vi "WAIT.vi"(7 "arguments":string[](array[string]), 9 "Reinit":bool, 10 "HMI to Control":T1, 11 "SensorInputData":T2) -> (1 "Done":bool, 2 "SensorInputDataOut":T2, 3 "HMI to Control Out":T1)   [LabVIEW 2015]
uses:
  Typedefs/SensorInputData.ctl
  Typedefs/HMI_to_Control.ctl
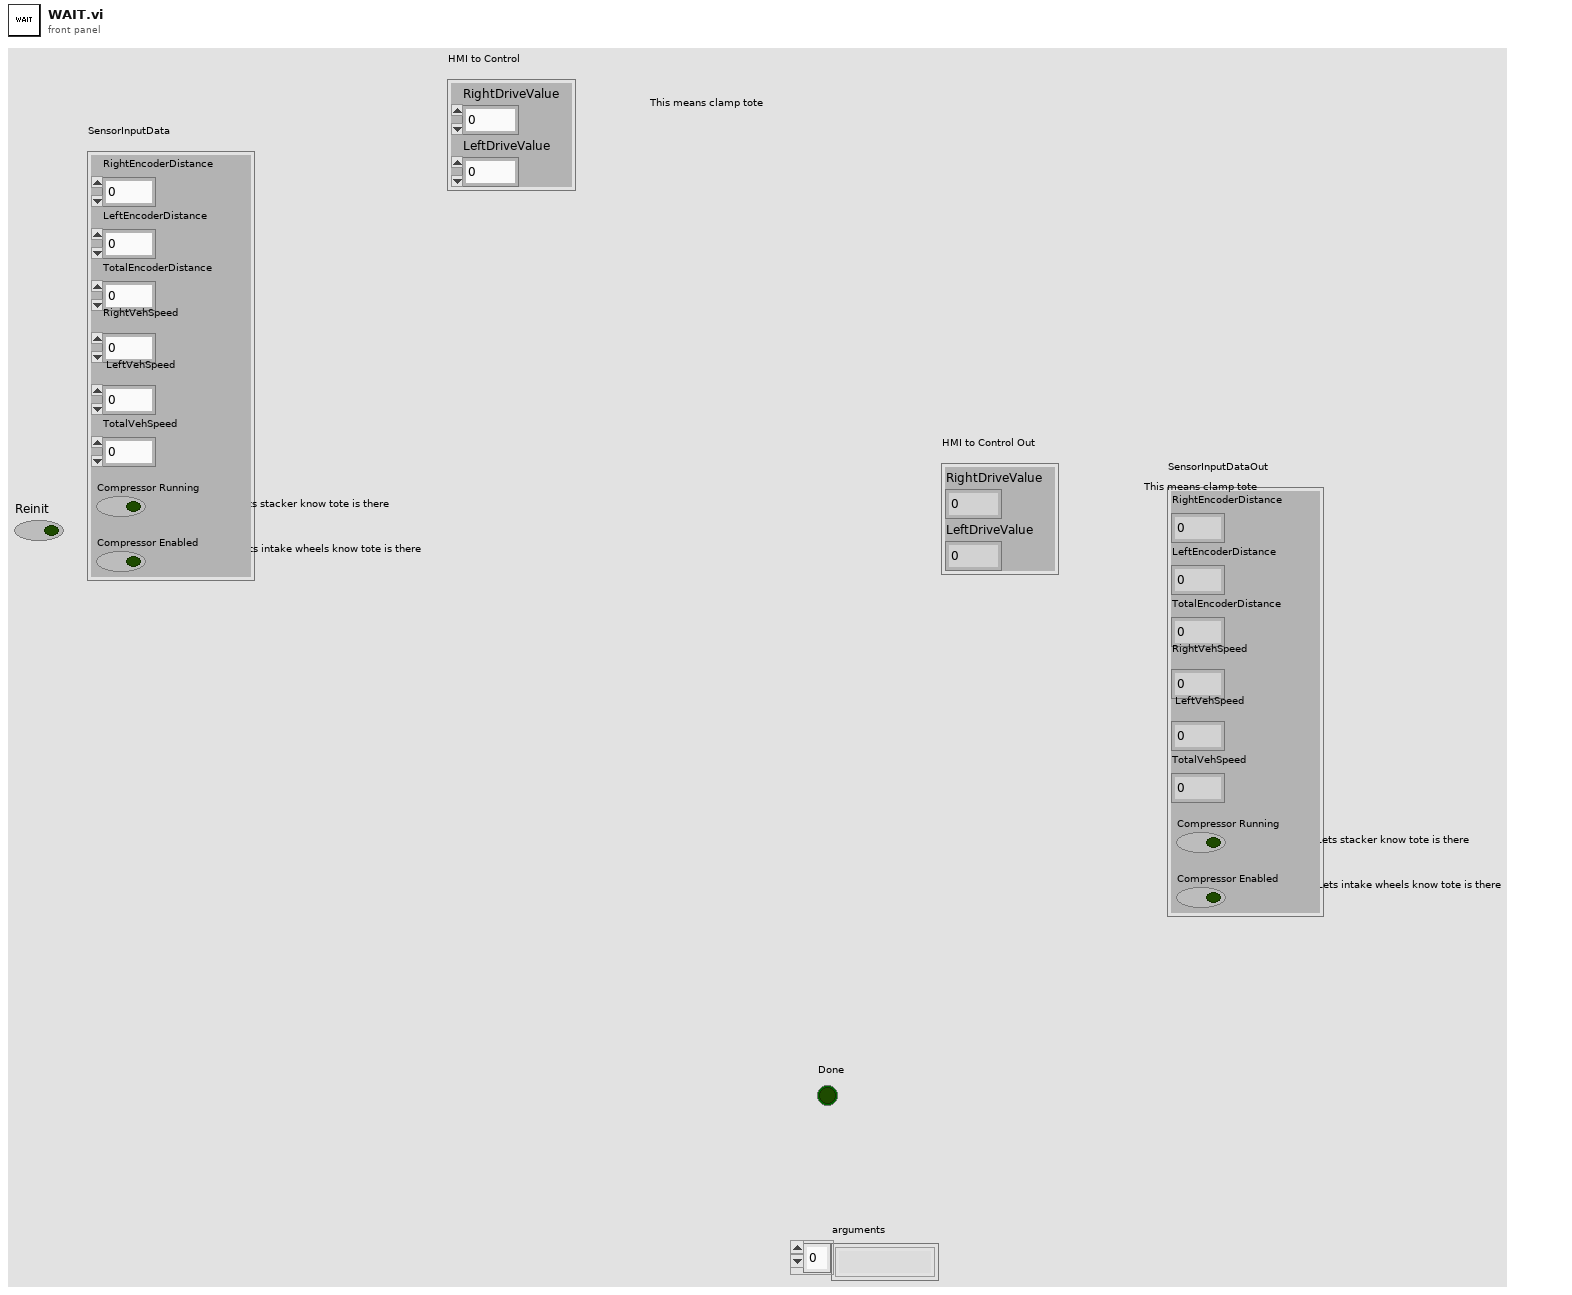
[diagram p1: front panel]
types:
  T1 = typedef "HMI_to_Control.ctl" = cluster{"RightDriveValue":dbl, "LeftDriveValue":dbl}
  T2 = typedef "SensorInputData.ctl" = cluster{"RightEncoderDistance":dbl, "LeftEncoderDistance":dbl, "TotalEncoderDistance":dbl, "RightVehSpeed":dbl, "LeftVehSpeed":dbl, "TotalVehSpeed":dbl, "Compressor Running":bool, "Compressor Enabled":bool}
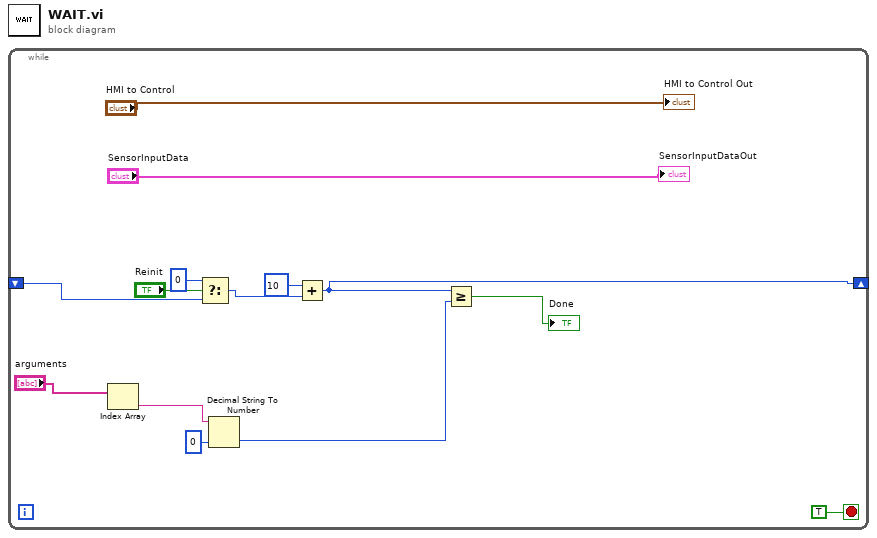
[diagram p0: block diagram]
diagram:
  n1 = while {
    shift-right: [w8] -> _
    shift-left: _ -> [w10]
    stop <- TRUE stop-if-true
    n2 = Index Array(array="arguments") -> (element=w13:string)  [unwired: 1 in]
    n3 = Select(t=0, s="Reinit", f=w10) -> (s? t:f=w9:i32)
    n4 = Decimal String To Number(string=w13, default (0L)=0 ("default (0 I32)")) -> (number=w6:i32)  [unwired: 1 in, 1 out]
    n5 = Add(x=10, y=w9) -> (x+y=w8:i32)
    n6 = Greater Or Equal?(x=w8, y=w6) -> (x >= y?=→"Done":bool)
    "SensorInputDataOut" <- "SensorInputData"
    "HMI to Control Out" <- "HMI to Control"
  }
